vi "Power data.vi"(6 "end":dbl=1.0 format="%.2p", 7 "start":dbl=0.001 format="%.2p", 8 "a":dbl=1.0 format="%0.2f", 9 "b":dbl=3.0 format="%0.2f", 10 "Number of points":i32=15, 11 "noise":dbl=1.0 format="%0.2f") -> (2 "X Array":dbl[](array[numeric]), 3 "Y Array":dbl[](array[numeric]))   [LabVIEW 2023]
doc: "Creates a set of power data according to the model y = a*(b^x)."
uses:
  <vilib>/Analysis/1siggen.llb/Ramp Pattern by Samples.vi
  <vilib>/Analysis/NI_AALBase.lvlib
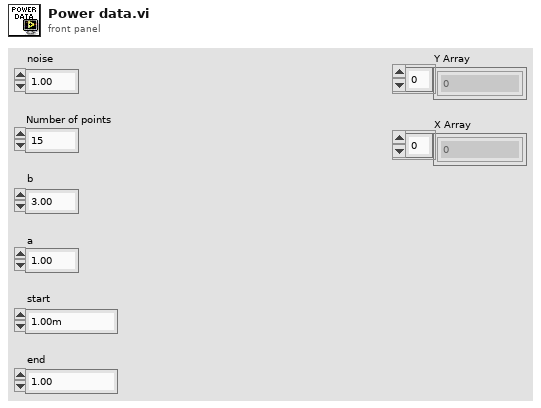
[diagram p1: front panel]
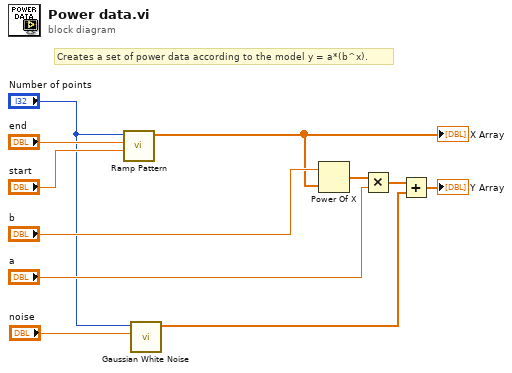
[diagram p0: block diagram]
diagram:
  # "Creates a set of power data according to the model y = a*(b^x)."
  n1 = call-poly <vilib>:"Ramp Pattern.vi"("start"="start", "end"="end", "samples"="Number of points") -> ("Ramp Pattern"=w6:dbl[])  [unwired: 7 in, 1 out]
  "X Array" <- w6
  n2 = call <vilib>:"Gaussian White Noise.vi"("standard deviation"="noise", "samples"="Number of points") -> ("Gaussian noise pattern"=w1:dbl[])  [unwired: 8 in, 1 out]
  n3 = Power Of X(1:w6, 2:"b") -> (0:w9:dbl[])
  n4 = Multiply(x=w9, y="a") -> (x*y=w11:dbl[])
  n5 = Add(x=w11, y=w1) -> (x+y=→"Y Array":dbl[])
